vi "RT_DataMonitor.vi"() -> ()   [LabVIEW 2010]
uses:
  <vilib>/Utility/error.llb/DialogType.ctl
  <vilib>/Pansino Software/LabVIEW Architecture/PSARC_Queue Management.llb/PSARC_Queue Create_Single.vi
  <vilib>/Pansino Software/LabVIEW Architecture/PSARC_Queue Management.llb/PSARC_Queue Destroy_Single.vi
  <vilib>/Pansino Software/LabVIEW Architecture/PSARC_Queue Management.llb/PSARC_Queue Valid.vi
  <vilib>/Pansino Software/LabVIEW Architecture/PSARC_Queue Management.llb/PSARC_Queue Remove Element.vi
panel:
  in  "Parameter":cluster{"Event":string, "Variant":variant}
  out "Error Report":string
  out "Current State":string
  in  "Exit Program":bool
  # "/* -------- Notes for All Users -------- */\nRecommand : \n[1].Display Setting Resolution -> 1440x900\n[2].Read Arch Notes First.\n[3].Make A Call When You Are In Trouble.\n\nTeam Members:\nPansino Soft,Pansino SDMA\n\nCopyright@2010 Pansino.Beijing\n\nVersion Number: 2010"
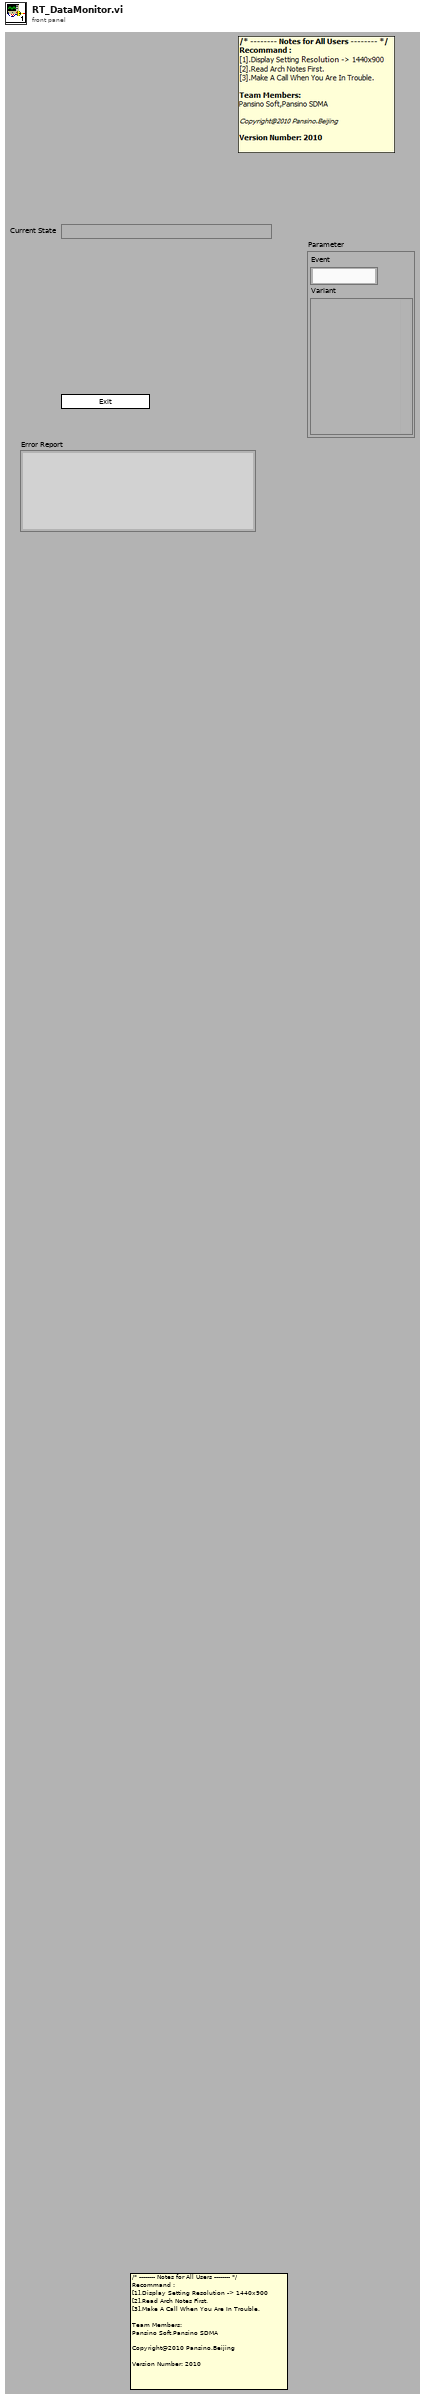
[diagram p1: front panel]
types:
  T1 = cluster{"Error":errorcluster, "VIRef":refnum<vi>, "Exit":bool, "System Path":cluster{"Data Folder Path":path}, "Q-Local":cluster{"Q-Local Name":string, "Q-Local Order":string, "Q-Local Data":variant}, "Q-HighLevel":cluster{"Q-HighLevel Name":string, "Q-HighLevel Order":string, "Q-HighLevel Data":variant}, "writer endpoint":refnum<k21>}
  T2 = typedef "DialogType.ctl" = u16
  T3 = cluster{"Q-HighLevel Order":string, "Q-HighLevel Data":variant}
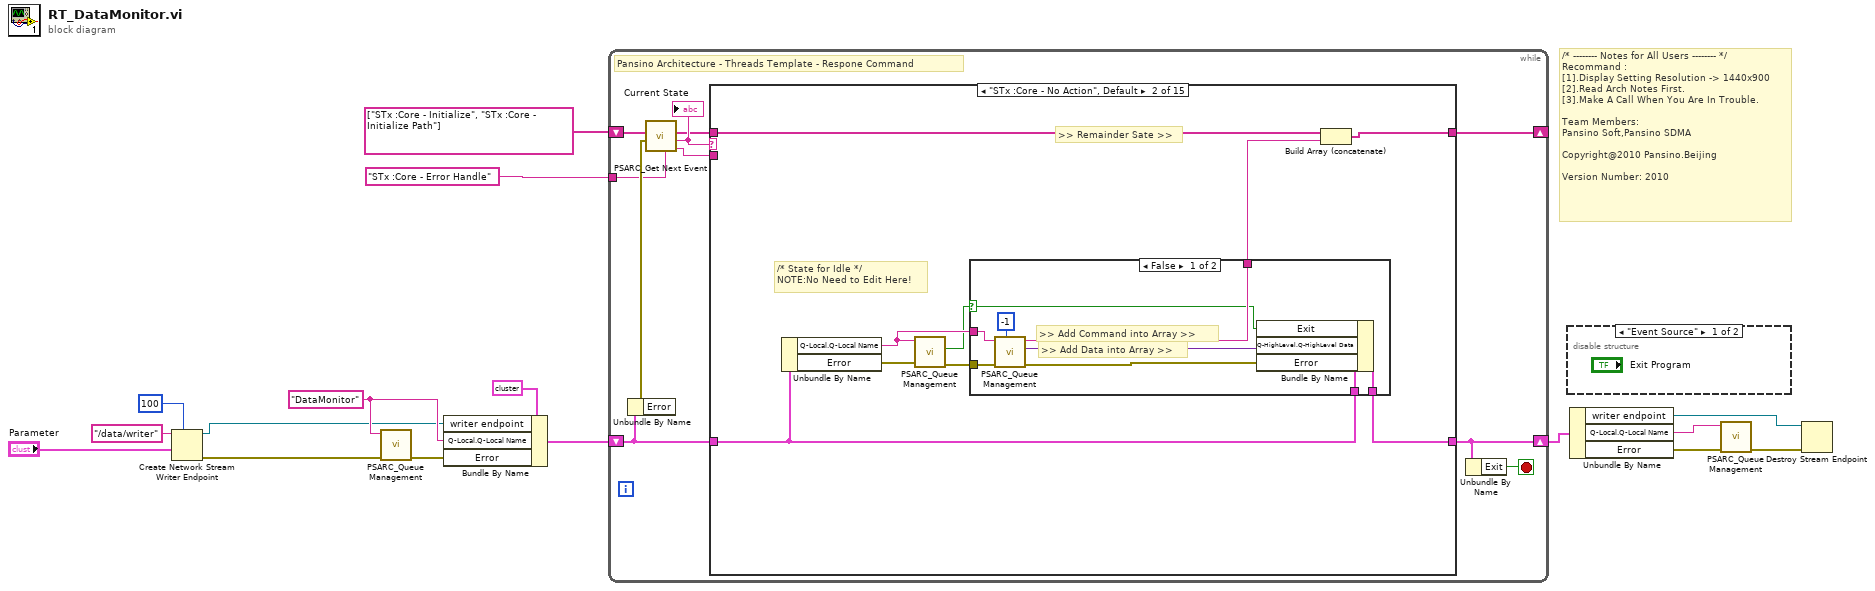
[diagram p0: block diagram]
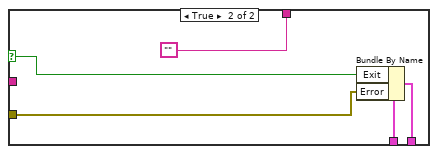
[diagram p4: hidden frame]
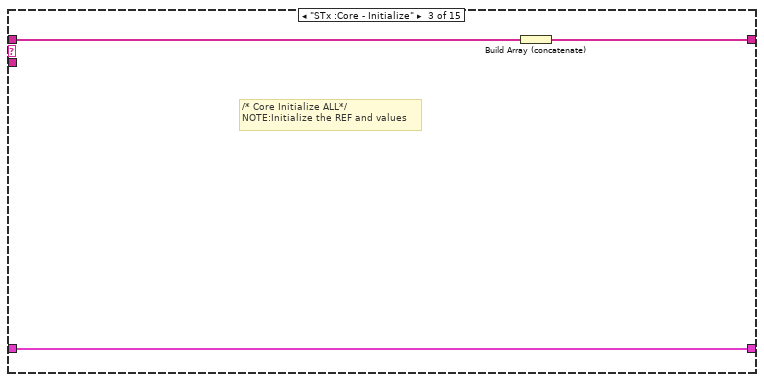
[diagram p5: hidden frame]
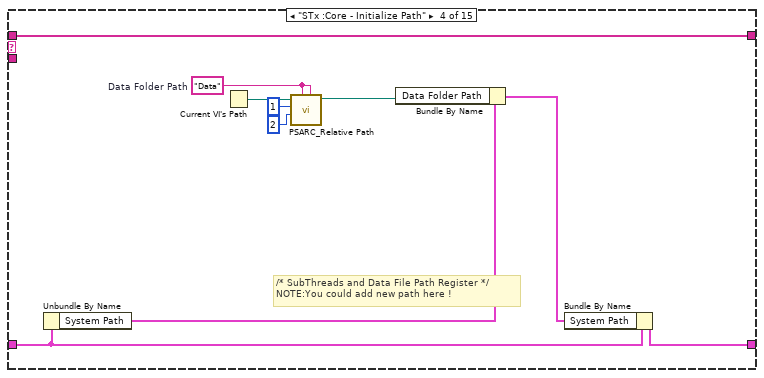
[diagram p6: hidden frame]
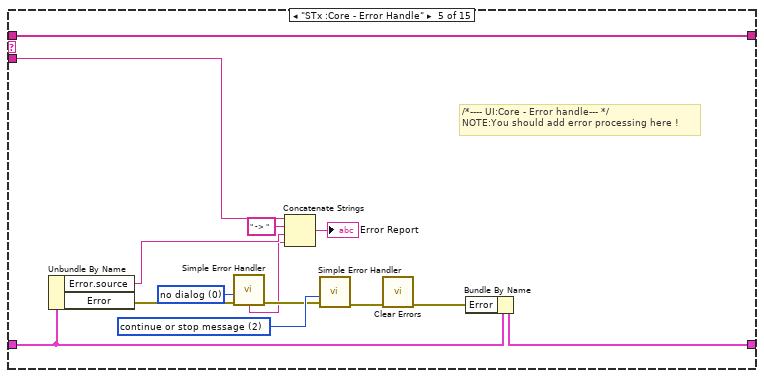
[diagram p7: hidden frame]
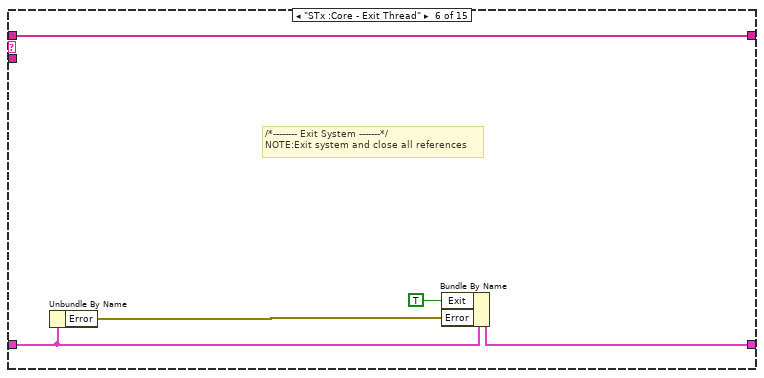
[diagram p8: hidden frame]
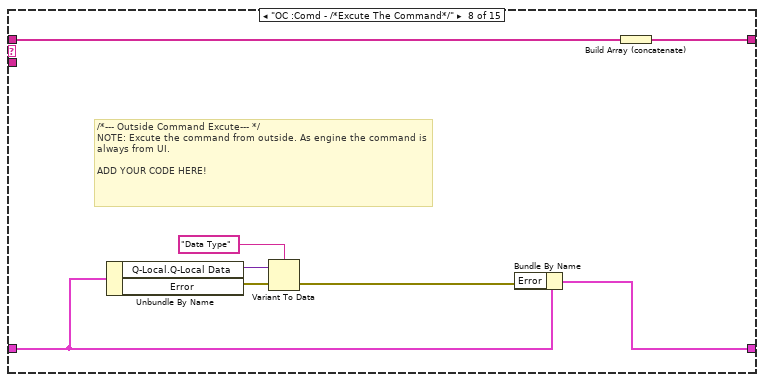
[diagram p10: hidden frame]
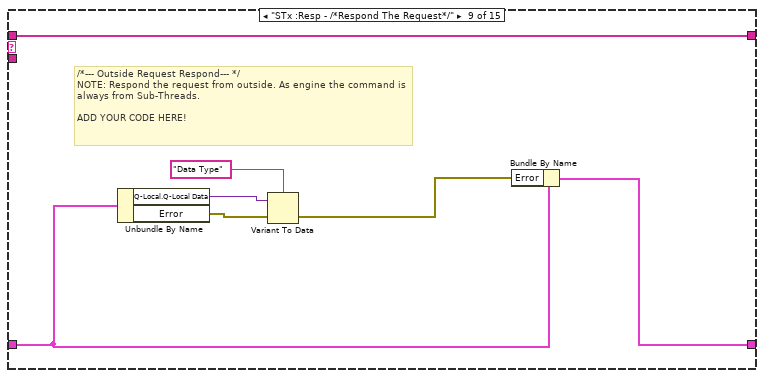
[diagram p11: hidden frame]
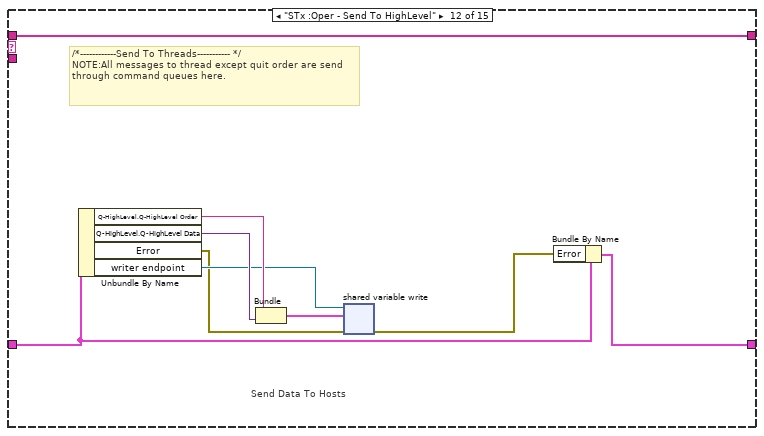
[diagram p14: hidden frame]
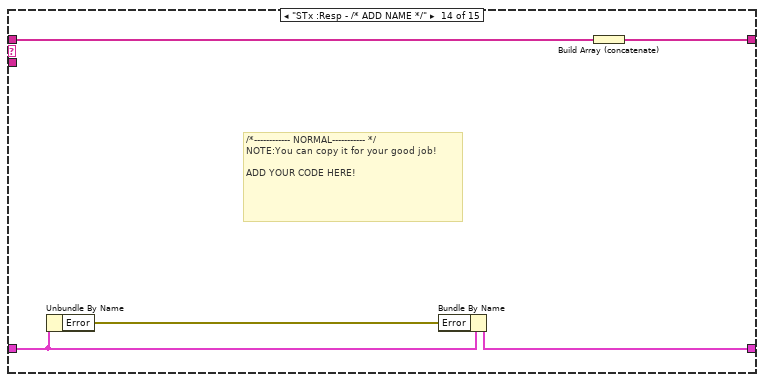
[diagram p16: hidden frame]
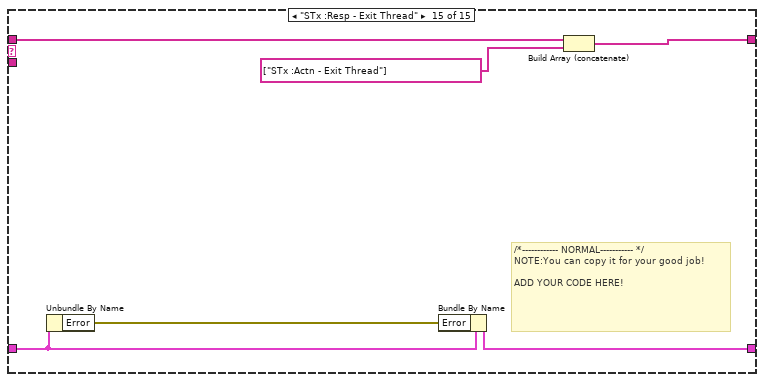
[diagram p17: hidden frame]
diagram:
  w4 = "DataMonitor" ("Queue Name")
  # "/* -------- Notes for All Users -------- */\nRecommand : \n[1].Display Setting Resolution -> 1440x900\n[2].Read Arch Notes First.\n[3].Make A Call When You Are In Trouble.\n\nTeam Members:\nPansino Soft,Pansino SDMA\n\nCopyright@2010 Pansino.Beijing\n\nVersion Number: 2010"
  n1 = Create Network Stream Writer Endpoint(7:100 ("writer buffer size"), 9:"Parameter", 11:"/data/writer" ("writer name")) -> (0:w2:errorcluster, 3:w3:refnum<k21>)  [unwired: 3 in]
  n2 = call-poly <vilib>:"PSARC_Queue Management.vi"("error in (no error)"=w2, "Queue Name"=w4) -> ("error out"=w1:errorcluster)  [unwired: 8 in, 1 out]
  n3 = Bundle By Name(cluster=T1 {"Error"={"status"=FALSE, "code"=0, "source"=""}, "VIRef"=refnum, "Exit"=FALSE, "System Path"={"Data Folder Path"=path ""}, "Q-Local"={"Q-Local Name"="", "Q-Local Order"="", "Q-Local Data"=variant}, "Q-HighLevel"={"Q-HighLevel Name"="", "Q-HighLevel Order"="", "Q-HighLevel Data"=variant}, "writer endpoint"=""} ("TempVariable"), "writer endpoint"=w3, "Q-Local.Q-Local Name"=w4, "Error"=w1) -> (w13:T1)
  n4 = while {
    shift-right: [w20] -> w16
    shift-left: w13 -> [w22]
    shift-right: [w23] -> _
    shift-left: string[] ["STx :Core - Initialize", "STx :Core - Initialize Path"] -> [w26]
    tunnel: "STx :Core - Error Handle" ("Error Handle") -> [w18]
    stop <- w19 stop-if-true
    # "Pansino Architecture - Threads Template - Respone Command"
    n5 = Unbundle By Name(w22) -> ("Error"=w21:errorcluster)
    n6 = call <vilib>:"PSARC_Get Next Event.vi"("Error Handle"=w18, "error in (no error)"=w21, "event queue in"=w26) -> ("prev event"=w17:string, "next event"=w25:string, "event queue out"=w24:string[])  [unwired: 3 in]
    "Current State" <- w25
    n7 = case shown="\"STx :Core - No Action\", Default" w25 {
      tunnel: w22 -> [w27 w37 w53 w62 w76 w80 w84 w90 w99 w101 w103 w112 w114 w119 w125]
      tunnel: w24 -> [w28 w35 w54 w64 w78 w83 w85 w93 w100 w102 w104 w113 w115 w117 w123]
      tunnel: [w28 w34 w52 w64 w78 w83 w85 w91 w100 w102 w104 w113 w115 w116 w122] -> w23
      tunnel: [w27 w36 w53 w63 w77 w81 w84 w92 w98 w101 w103 w111 w114 w118 w124] -> w20
      tunnel: w17 -> [_ _ _ _ w69 _ _ _ _ _ _ _ _ _ _]
      frame "----------Core Status----------" {
        # "/----------* System Core Part *----------/\nNOTE:This part included the normal operations in all programs, such as initial, error handle, exit and so on."
      }
      frame "STx :Core - No Action", Default {
        # "/* State for Idle */\nNOTE:No Need to Edit Here!"
        # ">> Remainder Sate >>"
        n8 = Unbundle By Name(w37) -> ("Q-Local.Q-Local Name"=w32:string, "Error"=w31:errorcluster)
        n9 = call-poly <vilib>:"PSARC_Queue Management.vi"("error in (no error)"=w31, "Queue Name(unamed)"=w32) -> ("error out"=w30:errorcluster, "Not a queue?"=w29:bool)  [unwired: 8 in]
        n10 = case shown="False" w29 {
          selector: w29 -> [w38 w49]
          tunnel: w37 -> [w44 w50]
          tunnel: [w43 w47] -> w36
          tunnel: [w42 "" ("Event")] -> w33
          tunnel: w32 -> [w40 _]
          tunnel: w30 -> [w39 w48]
          frame False {
            # ">> Add Data into Array >>"
            # ">> Add Command into Array >>"
            n11 = call-poly <vilib>:"PSARC_Queue Management.vi"("Time out(-1)_queue out"=-1, "error in (no error)"=w39, "Queue Name(unamed)"=w40) -> ("error out"=w46:errorcluster, "Data"=w45:variant, "Event"=w42:string)  [unwired: 5 in, 1 out]
            n12 = Bundle By Name(cluster=w44, "Exit"=w38, "Q-HighLevel.Q-HighLevel Data"=w45, "Error"=w46) -> (w43:T1)
          }
          frame True {
            n13 = Bundle By Name(cluster=w50, "Exit"=w49, "Error"=w48) -> (w47:T1)
          }
        }
        n14 = Build Array (concatenate)(w35, w33) -> (w34:string[])
      }
      frame "STx :Core - Initialize" {
        # "/* Core Initialize ALL*/\nNOTE:Initialize the REF and values"
        n15 = Build Array (concatenate)(w54) -> (w52:string[])
      }
      frame "STx :Core - Initialize Path" {
        w57 = "Data"  # Data Folder Path
        # "/* SubThreads and Data File Path Register */\nNOTE:You could add new path here !"
        n16 = Unbundle By Name(w62) -> ("System Path"=w56:cluster{"Data Folder Path":path})
        n17 = Current VI's Path() -> (path=w58:path)
        n18 = call <vilib>:"PSARC_Relative Path.vi"("Development Relative Path"=w57, "Run Time relative path"=w57, "Run-Time File Depth"=2, "Development File Depth"=1, "Root Path"=w58) -> ("Relative Path"=w61:path)  [unwired: 5 in, 1 out]
        n19 = Bundle By Name(cluster=w56, "Data Folder Path"=w61) -> (w55:cluster{"Data Folder Path":path})
        n20 = Bundle By Name(cluster=w62, "System Path"=w55) -> (w63:T1)
      }
      frame "STx :Core - Error Handle" {
        w70 = T2 0 items=["no dialog", "OK message", "continue or stop message", "OK message + warnings", "continue/stop + warnings"] ("type of dialog (OK msg:1)")
        w73 = T2 2 items=["no dialog", "OK message", "continue or stop message", "OK message + warnings", "continue/stop + warnings"] ("type of dialog (OK msg:1)")
        # "/*---- UI:Core - Error handle--- */\nNOTE:You should add error processing here !"
        n21 = Unbundle By Name(w76) -> ("Error.source"=w67:string, "Error"=w72:errorcluster)
        n22 = call <vilib>:"Simple Error Handler.vi"("type of dialog (OK msg:1)"=w70, "error in (no error)"=w72) -> ("error out"=w71:errorcluster, "message"=w66:string)  [unwired: 3 in, 3 out]
        n23 = Concatenate Strings(w69, " -> " ("字符串"), w67, w66) -> (→"Error Report":string)
        n24 = call <vilib>:"Simple Error Handler.vi"("type of dialog (OK msg:1)"=w73, "error in (no error)"=w71) -> ("error out"=w75:errorcluster)  [unwired: 3 in, 4 out]
        n25 = call <vilib>:"Clear Errors.vi"("error in (no error)"=w75) -> ("error out"=w74:errorcluster)  [unwired: 6 in]
        n26 = Bundle By Name(cluster=w76, "Error"=w74) -> (w77:T1)
      }
      frame "STx :Core - Exit Thread" {
        # "/*-------- Exit System -------*/\nNOTE:Exit system and close all references"
        n27 = Unbundle By Name(w80) -> ("Error"=w82:errorcluster)
        n28 = Bundle By Name(cluster=w80, "Exit"=TRUE, "Error"=w82) -> (w81:T1)
      }
      frame "----------Send And Resp----------" {
        # "/----------* Send Order And Respond Part *----------/\nNOTE:This part included the queue operations, which is used to send datas and orders to dynamic threads."
      }
      frame "OC :Comd - /*Excute The Command*/" {
        # "/*--- Outside Command Excute--- */\nNOTE: Excute the command from outside. As engine the command is always from UI.\n\nADD YOUR CODE HERE!"
        n29 = Unbundle By Name(w90) -> ("Q-Local.Q-Local Data"=w89:variant, "Error"=w88:errorcluster)
        n30 = Variant To Data(error in=w88, Variant=w89, type="Data Type" ("Data Type")) -> (error out=w86:errorcluster)  [unwired: 1 out]
        n31 = Bundle By Name(cluster=w90, "Error"=w86) -> (w92:T1)
        n32 = Build Array (concatenate)(w93) -> (w91:string[])
      }
      frame "STx :Resp - /*Respond The Request*/" {
        # "/*--- Outside Request Respond--- */\nNOTE: Respond the request from outside. As engine the command is always from Sub-Threads.\n\nADD YOUR CODE HERE!"
        n33 = Unbundle By Name(w99) -> ("Q-Local.Q-Local Data"=w96:variant, "Error"=w97:errorcluster)
        n34 = Variant To Data(error in=w97, Variant=w96, type="Data Type" ("Data Type")) -> (error out=w95:errorcluster)  [unwired: 1 out]
        n35 = Bundle By Name(cluster=w99, "Error"=w95) -> (w98:T1)
      }
      frame "----------Actions----------" {
        # "/----------* Actions *----------/\nNOTE:This part included the ALL the actions."
      }
      frame "----------Operation----------" {
        # "/----------* Operation Part *----------/\nNOTE:This part included the user operations."
      }
      frame "STx :Oper - Send To HighLevel" {
        # "Send Data To Hosts"
        # "/*------------Send To Threads----------- */\nNOTE:All messages to thread except quit order are send through command queues here."
        n36 = Unbundle By Name(w112) -> ("Q-HighLevel.Q-HighLevel Order"=w108:string, "Q-HighLevel.Q-HighLevel Data"=w109:variant, "Error"=w106:errorcluster, "writer endpoint"=w107:refnum<k21>)
        n37 = Bundle("Q-HighLevel Order"=w108, "Q-HighLevel Data"=w109) -> (w110:T3)  [unwired: 1 in]
        n38 = shared-variable-write(w107, w106, w110) -> (w105:errorcluster)  [unwired: 1 in, 2 out]
        n39 = Bundle By Name(cluster=w112, "Error"=w105) -> (w111:T1)
      }
      frame "----------Respond Events----------" {
        # "/----------* Respond Order Part *----------/\nNOTE:This part included the operations from main queue, which is used to respond the dynamic threads."
      }
      frame "STx :Resp - /* ADD NAME */" {
        # "/*------------ NORMAL----------- */\nNOTE:You can copy it for your good job!\n\nADD YOUR CODE HERE!"
        n40 = Unbundle By Name(w119) -> ("Error"=w120:errorcluster)
        n41 = Bundle By Name(cluster=w119, "Error"=w120) -> (w118:T1)
        n42 = Build Array (concatenate)(w117) -> (w116:string[])
      }
      frame "STx :Resp - Exit Thread" {
        # "/*------------ NORMAL----------- */\nNOTE:You can copy it for your good job!\n\nADD YOUR CODE HERE!"
        n43 = Unbundle By Name(w125) -> ("Error"=w126:errorcluster)
        n44 = Bundle By Name(cluster=w125, "Error"=w126) -> (w124:T1)
        n45 = Build Array (concatenate)(w123, string[] ["STx :Actn - Exit Thread"] ("数组")) -> (w122:string[])
      }
    }
    n46 = Unbundle By Name(w20) -> ("Exit"=w19:bool)
  }
  n47 = disable-structure shown="\"Event Source\"" {
    frame condition #0 (active) {
    }
    frame condition #1 {
    }
  }
  n48 = Unbundle By Name(w16) -> ("writer endpoint"=w6:refnum<k21>, "Q-Local.Q-Local Name"=w14:string, "Error"=w15:errorcluster)
  n49 = call-poly <vilib>:"PSARC_Queue Management.vi"("error in (no error)"=w15, "Queue Name(unamed)"=w14) -> ("error out"=w5:errorcluster)  [unwired: 7 in, 2 out]
  n50 = Destroy Stream Endpoint(8:w5, 11:w6) -> ()  [unwired: 1 out]
